vi "Shutdown.vi"(8 "error in (no error)":errorcluster, 11 "Digital Delay Generator in":refnum<class "Digital Delay Generator.lvclass">) -> (0 "error out":errorcluster, 3 "Digital Delay Generator out":refnum<class "Digital Delay Generator.lvclass">)   [LabVIEW 2018, in "Digital Delay Generator.lvlib" / "Digital Delay Generator.lvclass"]
uses:
  Digital Delay Generator.lvclass
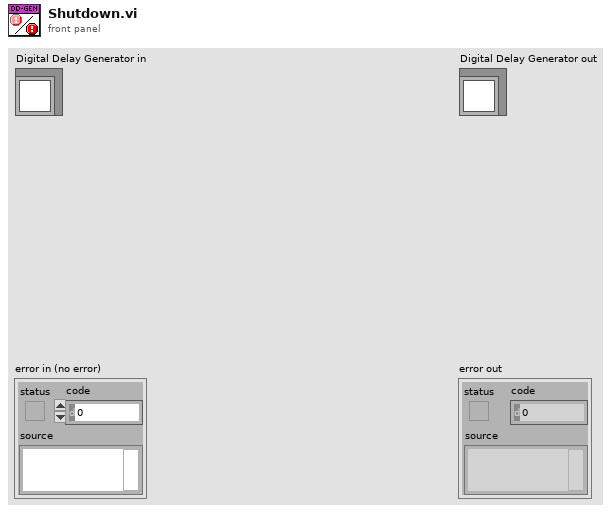
[diagram p1: front panel]
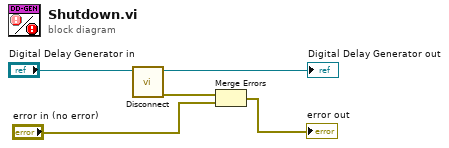
[diagram p0: block diagram]
diagram:
  n1 = call-dynamic "Disconnect.vi"("Digital Delay Generator in"="Digital Delay Generator in") -> ("error out"=w3:errorcluster, "Digital Delay Generator out"=→"Digital Delay Generator out":refnum<class "Digital Delay Generator.lvclass">)  [unwired: 9 in]
  n2 = Merge Errors(w3, "error in (no error)") -> (→"error out":errorcluster)
